vi "Galvo Module-continuous.vi"(7 "Action":T9(ring)=enum."calculate", 8 "error in (no error)":errorcluster, 10 "System Parameters":T1={"Optical Parameters"={"Obj. Focal Length [mm]"=45.0, "Scan Lens EFL[mm]"=60.0, "Tube Lens EFL[mm]"=180.0, "Galvo V Range (+/-)"=10.0, "Galvo Max Half Angle [Deg]"=19.0, "Max Galvo Range[%]"=0.0}, "Vibratome"={"Z Bottom [mm]"=0.0, "Pre Cut Dwell [s]"=0.0, "Blade Frequency [RPM]"=0, "Slice Speed [mm/s]"=0.0, "Post Cut Dwell [s]"=0.0, "Ramp Time [s]"=0.0, "Start X [mm]"=0.0, "Start Y [mm]"=0.0, "Slice Length [mm]"=0.0, "Slice Axis"=enum."Y Axis", "Controller VISA Ref"="COM4"}, "Table Stages"={"X Stage"={"Position"=0.0, "Is.Enabled?"=FALSE, "Is.Connected?"=FALSE, "Device SN"="45876539", "AccelerationMaximum"=0.0, "VelocityMaximum"=0.0, "Acceleration"=0.0, "Velocity"=0.0, "waitTimeout (ms)"=0, "Model"=enum."None", "Is.Homed?"=FALSE}, "Y Stage"={"Position"=0.0, "Is.Enabled?"=FALSE, "Is.Connected?"=FALSE, "Device SN"="45876539", "AccelerationMaximum"=0.0, "VelocityMaximum"=0.0, "Acceleration"=0.0, "Velocity"=0.0, "waitTimeout (ms)"=0, "Model"=enum."None", "Is.Homed?"=FALSE}, "Z Stage"={"Position"=0.0, "Is.Enabled?"=FALSE, "Is.Connected?"=FALSE, "Device SN"="45876539", "AccelerationMaximum"=0.0, "VelocityMaximum"=0.0, "Acceleration"=0.0, "Velocity"=0.0, "waitTimeout (ms)"=0, "Model"=enum."None", "Is.Homed?"=FALSE}}, "Imaging Parameter"={"Raster Scan Direction"=enum."Uni Directional", "Pixel Dwell Time [Clock Cycles]"=1, "Flyback Time [Clock Cycles]"=10, "XY Center [um]"={"X"=1.0, "Y"=1.0}, "Pixel Step Size [um]"=50.0, "XY Image Size"=enum."256 x 256", "Custom"=TRUE, "Custom Size"={"X"=10, "Y"=10}, "Line Averages"=1}} {"Imaging Parameter"."Line Averages" min=1 max=30 step=1; "Imaging Parameter"."Flyback Time [Clock Cycles]" max=10 step=1; "Imaging Parameter"."Pixel Step Size [um]" min=0.0 max=10.0 step=0.01; "Imaging Parameter"."Custom Size"."Y" min=1 max=30 step=1; "Imaging Parameter"."Custom Size"."X" min=1 max=30 step=1; "Imaging Parameter"."XY Center [um]"."Y" min=1.0 max=30.0 step=1.0; "Imaging Parameter"."XY Center [um]"."X" min=1.0 max=30.0 step=1.0; "Imaging Parameter"."Pixel Dwell Time [Clock Cycles]" max=10 step=1}, 11 "Galvo HW Parameters":T10={"Analog Out Channel"="Dev1/ao0", "Min Voltage"=-5.0, "Max Voltage"=5.0, "Pixel Clock Source"="OnboardClock", "Sample Rate"=1000.0, "Line Clock Out Ch"=""}) -> (0 "error out":errorcluster)   [LabVIEW 2018]
uses:
  Controls/System Parameters.ctl
  Controls/Optical Parameters.ctl
  Controls/Vibratome Parameters.ctl
  Controls/Translation Stage Parameters.ctl
  Hardware Mfg/Thorlabs Translation Stages/Controls/Translation Stage Cluster.ctl
  Controls/Translation Stage Types.ctl
  Controls/Imaging Parameters.ctl
  Controls/Scan Direction.ctl
  <vilib>/DAQmx/write.llb/DAQmx Write (Digital 1D U32 1Chan NSamp).vi
  <vilib>/DAQmx/write.llb/DAQmx Write (Analog 2D DBL NChan NSamp).vi
  <vilib>/DAQmx/create/channels.llb/DAQmx Create Channel (DO-Digital Output).vi
  <vilib>/DAQmx/configure/timing.llb/DAQmx Timing (Sample Clock).vi
  <vilib>/DAQmx/create/channels.llb/DAQmx Create Channel (AO-Voltage-Basic).vi
  <vilib>/DAQmx/miscellaneous.llb/DAQmx Fill In Error Info.vi
  <resource>/objmgr/daqmx.rc
panel:
  out "task done?":bool
  # "X"
  # "X"
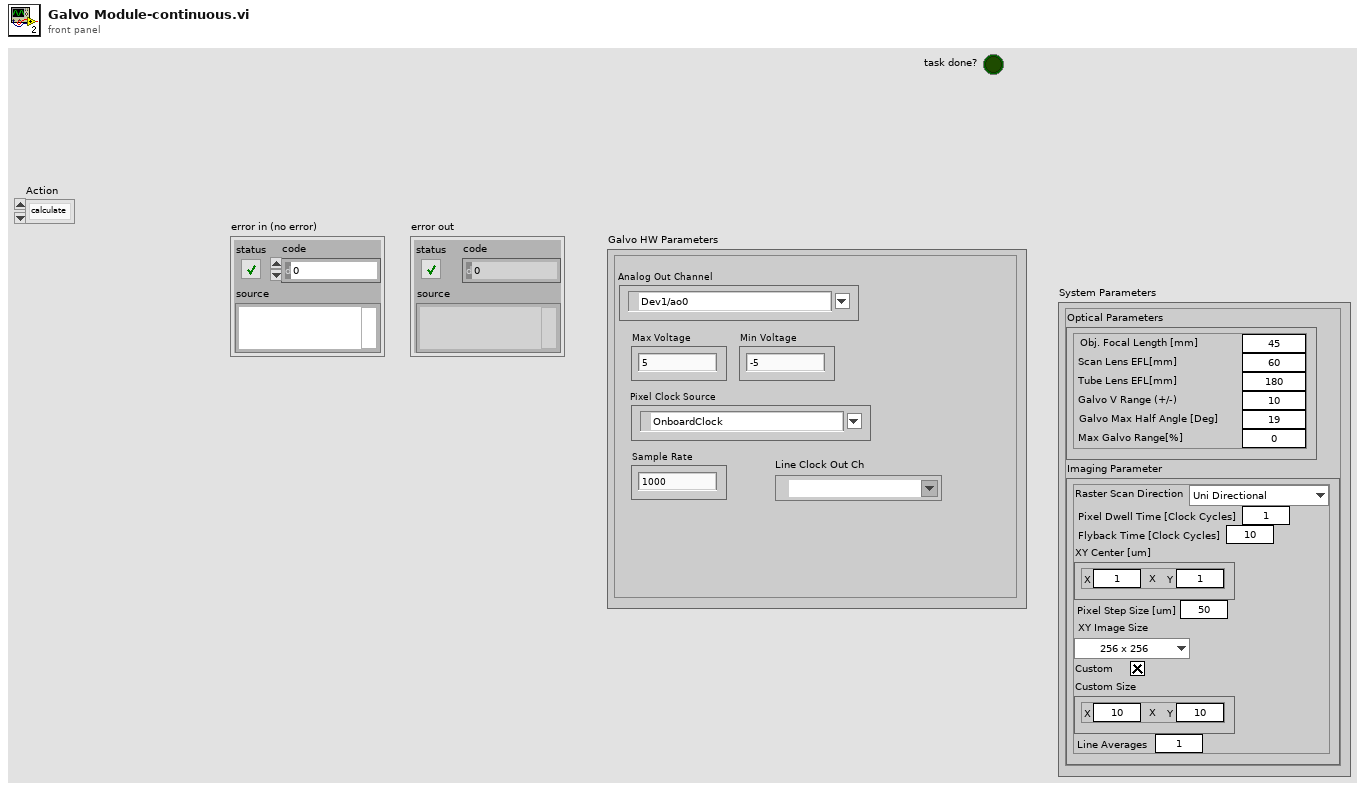
[diagram p1: front panel]
types:
  T1 = typedef "System Parameters.ctl" = cluster{"Optical Parameters":T2, "Vibratome":T3, "Table Stages":T4, "Imaging Parameter":T7}
  T2 = typedef "Optical Parameters.ctl" = cluster{"Obj. Focal Length [mm]":dbl, "Scan Lens EFL[mm]":dbl, "Tube Lens EFL[mm]":dbl, "Galvo V Range (+/-)":dbl, "Galvo Max Half Angle [Deg]":dbl, "Max Galvo Range[%]":dbl}
  T3 = typedef "Vibratome Parameters.ctl" = cluster{"Z Bottom [mm]":dbl, "Pre Cut Dwell [s]":dbl, "Blade Frequency [RPM]":u16, "Slice Speed [mm/s]":dbl, "Post Cut Dwell [s]":dbl, "Ramp Time [s]":dbl, "Start X [mm]":dbl, "Start Y [mm]":dbl, "Slice Length [mm]":dbl, "Slice Axis":enum16{"X Axis", "Y Axis", "Z Axis"}, "Controller VISA Ref":refnum<visa-resource-name>}
  T4 = typedef "Translation Stage Parameters.ctl" = cluster{"X Stage":T5, "Y Stage":T5, "Z Stage":T5}
  T5 = typedef "Translation Stage Cluster.ctl" = cluster{"Position":dbl, "Is.Enabled?":bool, "Is.Connected?":bool, "Device SN":string, "AccelerationMaximum":dbl, "VelocityMaximum":dbl, "Acceleration":dbl, "Velocity":dbl, "waitTimeout (ms)":i32, "Model":T6, "Is.Homed?":bool}
  T6 = typedef "Translation Stage Types.ctl" = enum16{"None", "Thorlabs LTS", "Thorlabs MLJ"}
  T7 = typedef "Imaging Parameters.ctl" = cluster{"Raster Scan Direction":T8, "Pixel Dwell Time [Clock Cycles]":u16, "Flyback Time [Clock Cycles]":u16, "XY Center [um]":cluster{"X":dbl, "Y":dbl}, "Pixel Step Size [um]":dbl, "XY Image Size":enum16{"32 x 32", "64 x 64", "128 x 128", "256 x 256", "512 x 512", "1024 x 1024", "2048 x 2048"}, "Custom":bool, "Custom Size":cluster{"X":u16, "Y":u16}, "Line Averages":u8}
  T8 = typedef "Scan Direction.ctl" = enum16{"Uni Directional", "Bi Directional", "None"}
  T9 = enum16{"Init", "Calc & Write Scan Pattern", "Start Galvo Task", "Is Task Done?", "Stop Galvo", "Uninit", "calculate"}
  T10 = cluster{"Analog Out Channel":tag, "Min Voltage":dbl, "Max Voltage":dbl, "Pixel Clock Source":tag, "Sample Rate":dbl, "Line Clock Out Ch":tag}
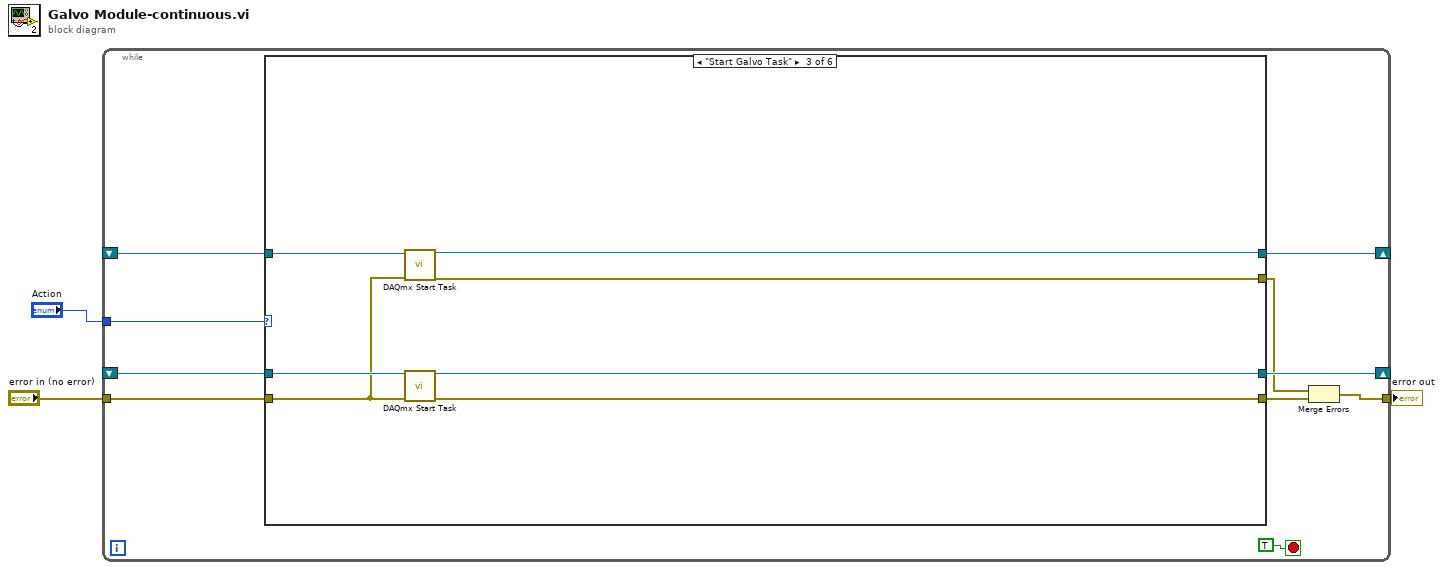
[diagram p0: block diagram]
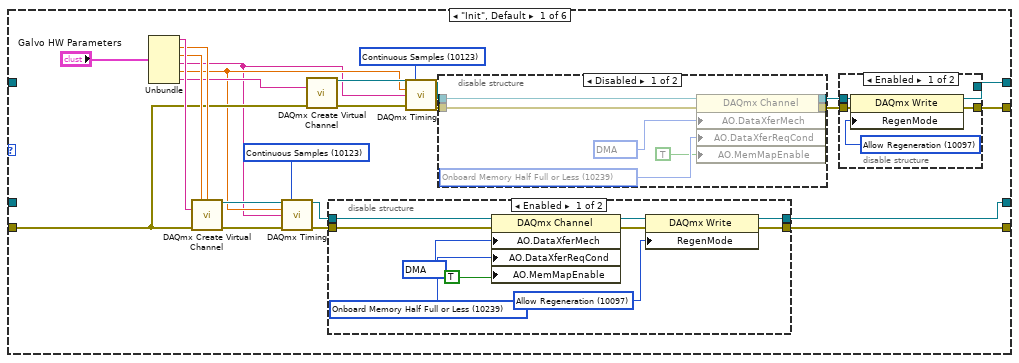
[diagram p2: hidden frame]
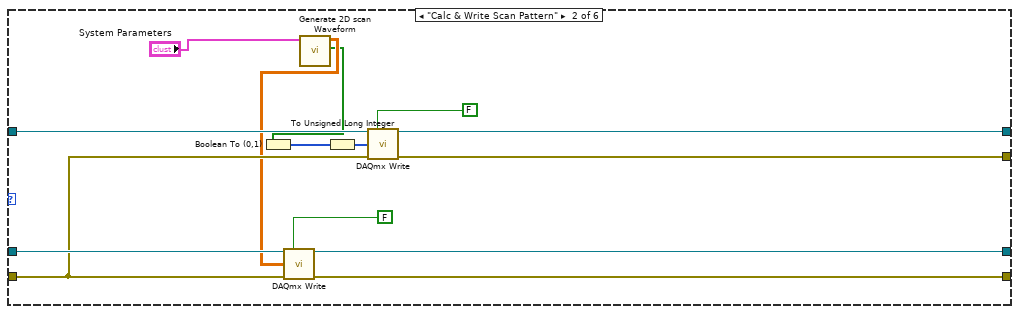
[diagram p6: hidden frame]
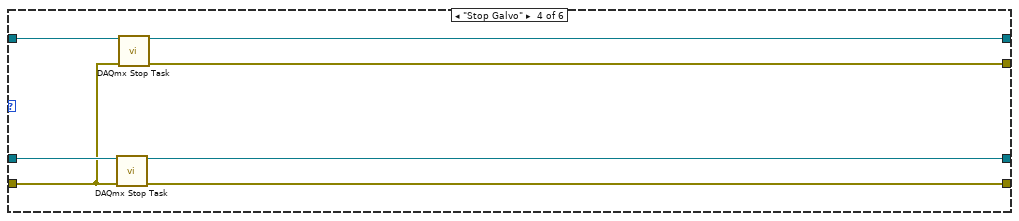
[diagram p7: hidden frame]
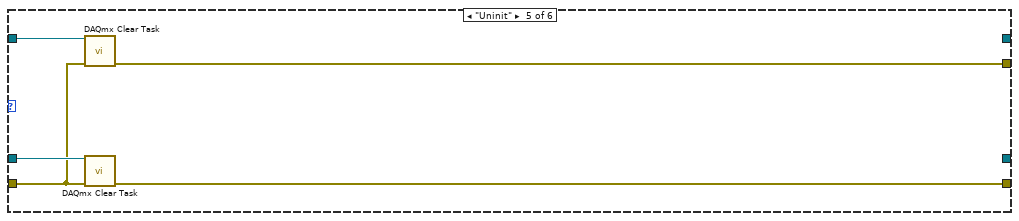
[diagram p8: hidden frame]
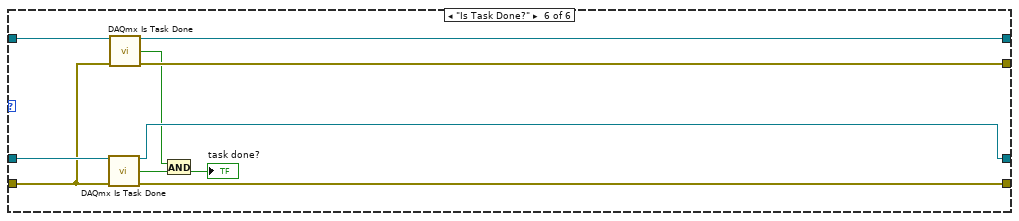
[diagram p9: hidden frame]
diagram:
  n1 = while {
    tunnel: "Action" -> [w13]
    shift-right: [w12] -> _
    shift-left: _ -> [w11]
    tunnel: [w7] -> w2
    tunnel: "error in (no error)" -> [w9]
    shift-right: [w5] -> _
    shift-left: _ -> [w4]
    stop <- TRUE stop-if-true
    n2 = case shown="\"Start Galvo Task\"" w13 {
      tunnel: [w30 w70 w85 w92 _ w106] -> w12
      tunnel: w11 -> [_ w79 w86 w93 w98 w108]
      tunnel: [w31 w71 w84 w91 w97 w107] -> w10
      tunnel: w9 -> [w26 w76 w83 w90 w94 w103]
      tunnel: [w18 w75 w80 w87 w96 w102] -> w6
      tunnel: [w17 w73 w81 w88 _ w99] -> w5
      tunnel: w4 -> [_ w72 w82 w89 w95 w104]
      frame "Init", Default {
        w15 = 10123 items=["Finite Samples"=10178, "Continuous Samples"=10123, "Hardware Timed Single Point"=12522] ("sample mode")
        w16 = 10123 items=["Finite Samples"=10178, "Continuous Samples"=10123, "Hardware Timed Single Point"=12522] ("sample mode")
        n3 = Unbundle("Galvo HW Parameters") -> ("Analog Out Channel"=w35:tag, "Min Voltage"=w34:dbl, "Max Voltage"=w33:dbl, "Pixel Clock Source"=w14:tag, "Sample Rate"=w23:dbl, "Line Clock Out Ch"=w29:tag)
        n4 = call-poly <vilib>:"DAQmx Create Virtual Channel.vi"("maximum value"=w33, "minimum value"=w34, "physical channels"=w35, "error in"=w26) -> ("task out"=w28:refnum<k21>, "error out"=w27:errorcluster)  [unwired: 10 in]
        n5 = call-poly <vilib>:"DAQmx Timing.vi"("task/channels in"=w28, "sample mode"=w15, "rate"=w23, "source"=w14, "error in"=w27) -> ("task out"=w32:refnum<k21>, "error out"=w37:errorcluster)  [unwired: 9 in]
        n6 = call-poly <vilib>:"DAQmx Create Virtual Channel.vi"("lines"=w29, "error in"=w26) -> ("task out"=w24:refnum<k21>, "error out"=w25:errorcluster)  [unwired: 12 in]
        n7 = disable-structure shown="Enabled" {
          disable-tunnel: w37 -> [w54 w55]
          disable-tunnel: w32 -> [w52 w56]
          disable-tunnel: [w48 w55] -> w31
          disable-tunnel: [w45 w56] -> w30
          frame Enabled {
            w46 = 10097 items=["Allow Regeneration"=10097, "Do Not Allow Regeneration"=10158] ("RegenMode")
            w50 = 10239 items=["Onboard Memory Empty"=10235, "Onboard Memory Half Full or Less"=10239, "Onboard Memory Less than Full"=10242] ("AO.DataXferReqCond")
            w51 = 10054 items=["DMA"=10054, "Interrupts"=10204, "Programmed I/O"=10264, "USB Bulk"=12590] ("AO.DataXferMech")
            n8 = property class="DAQmx Channel"(reference=w52, error in=w54, "AO.DataXferMech"=w51, "AO.DataXferReqCond"=w50, "AO.MemMapEnable"=TRUE) -> (reference out=w47:refnum<k21>, error out=w53:errorcluster)
            n9 = property class="DAQmx Write"(reference=w47, error in=w53, "RegenMode"=w46) -> (reference out=w45:refnum<k21>, error out=w48:errorcluster)
          }
          frame Disabled {
          }
        }
        n10 = call-poly <vilib>:"DAQmx Timing.vi"("task/channels in"=w24, "sample mode"=w16, "rate"=w23, "source"=w14, "error in"=w25) -> ("task out"=w19:refnum<k21>, "error out"=w20:errorcluster)  [unwired: 9 in]
        n11 = disable-structure shown="Disabled" {
          disable-tunnel: [w63 w64] -> w22
          disable-tunnel: [w62 w65] -> w21
          disable-tunnel: w20 -> [w58 w65]
          disable-tunnel: w19 -> [w57 w64]
          frame Disabled {
            w60 = 10239 items=["Onboard Memory Empty"=10235, "Onboard Memory Half Full or Less"=10239, "Onboard Memory Less than Full"=10242] ("AO.DataXferReqCond")
            w61 = 10054 items=["DMA"=10054, "Interrupts"=10204, "Programmed I/O"=10264, "USB Bulk"=12590] ("AO.DataXferMech")
            n12 = property class="DAQmx Channel"(reference=w57, error in=w58, "AO.DataXferMech"=w61, "AO.DataXferReqCond"=w60, "AO.MemMapEnable"=TRUE) -> (reference out=w63:refnum<k21>, error out=w62:errorcluster)
          }
          frame Enabled {
          }
        }
        n13 = disable-structure shown="Enabled" {
          disable-tunnel: w22 -> [w42 w44]
          disable-tunnel: w21 -> [w41 w43]
          disable-tunnel: [w39 w43] -> w18
          disable-tunnel: [w38 w44] -> w17
          frame Enabled {
            w40 = 10097 items=["Allow Regeneration"=10097, "Do Not Allow Regeneration"=10158] ("RegenMode")
            n14 = property class="DAQmx Write"(reference=w42, error in=w41, "RegenMode"=w40) -> (reference out=w38:refnum<k21>, error out=w39:errorcluster)
          }
          frame Disabled {
          }
        }
      }
      frame "Calc & Write Scan Pattern" {
        n15 = call "Generate 2D scan Waveform.vi"("System Parameters [In]"="System Parameters") -> ("Digital Line Acq"=w68:bool[], "XY"=w69:dbl[][])  [unwired: 5 in, 4 out]
        n16 = Boolean To (0,1)(Boolean=w68) -> (0, 1=w77:i16[])
        n17 = call-poly <vilib>:"DAQmx Write.vi"("task/channels in"=w79, "auto start"=FALSE, "data"=w69, "error in"=w76) -> ("task out"=w70:refnum<k21>, "error out"=w71:errorcluster)  [unwired: 9 in, 1 out]
        n18 = To Unsigned Long Integer(number=w77) -> (unsigned 32bit integer=w67:u32[])
        n19 = call-poly <vilib>:"DAQmx Write.vi"("task/channels in"=w72, "auto start"=FALSE, "data"=w67, "error in"=w76) -> ("task out"=w73:refnum<k21>, "error out"=w75:errorcluster)  [unwired: 9 in, 1 out]
      }
      frame "Start Galvo Task" {
        n20 = call <vilib>:"DAQmx Start Task.vi"("task/channels in"=w82, "error in"=w83) -> ("task out"=w81:refnum<k21>, "error out"=w80:errorcluster)  [unwired: 12 in]
        n21 = call <vilib>:"DAQmx Start Task.vi"("task/channels in"=w86, "error in"=w83) -> ("task out"=w85:refnum<k21>, "error out"=w84:errorcluster)  [unwired: 12 in]
      }
      frame "Stop Galvo" {
        n22 = call <vilib>:"DAQmx Stop Task.vi"("task/channels in"=w93, "error in"=w90) -> ("task out"=w92:refnum<k21>, "error out"=w91:errorcluster)  [unwired: 12 in]
        n23 = call <vilib>:"DAQmx Stop Task.vi"("task/channels in"=w89, "error in"=w90) -> ("task out"=w88:refnum<k21>, "error out"=w87:errorcluster)  [unwired: 12 in]
      }
      frame "Uninit" {
        n24 = call <vilib>:"DAQmx Clear Task.vi"("task in"=w95, "error in"=w94) -> ("error out"=w96:errorcluster)  [unwired: 13 in]
        n25 = call <vilib>:"DAQmx Clear Task.vi"("task in"=w98, "error in"=w94) -> ("error out"=w97:errorcluster)  [unwired: 13 in]
      }
      frame "Is Task Done?" {
        n26 = call <vilib>:"DAQmx Is Task Done.vi"("task/channels in"=w108, "error in"=w103) -> ("task out"=w106:refnum<k21>, "task done?"=w105:bool, "error out"=w107:errorcluster)  [unwired: 11 in]
        n27 = call <vilib>:"DAQmx Is Task Done.vi"("task/channels in"=w104, "error in"=w103) -> ("task out"=w99:refnum<k21>, "task done?"=w100:bool, "error out"=w102:errorcluster)  [unwired: 11 in]
        n28 = And(x=w100, y=w105) -> (x .and. y?=→"task done?":bool)
      }
    }
    n29 = Merge Errors(w6, w10) -> (w7:errorcluster)
  }
  "error out" <- w2
